vi "Set Event Stop Result_Info.vi"(8 "error in (no error)":errorcluster caption="entrée d'erreur (pas d'erreur)", 10 "Class Popup Result_Info":refnum<user-event>, 11 "Class Popup Result_Info (Virtual) en entrée":refnum<class "Class Popup Result_Info (Virtual).lvclass">) -> (0 "error out":errorcluster caption="sortie d'erreur", 3 "Class Popup Result_Info (Virtual) en sortie":refnum<class "Class Popup Result_Info (Virtual).lvclass">)   [LabVIEW 2020, in "Library Instrument & Equipement.lvlib" / "Library Popup.lvlib" / "Class Popup Result_Info (Virtual).lvclass"]
uses:
  Class Popup Result_Info (Virtual).lvclass
  Class Popup Result_Info (Virtual).lvclass/Class Popup Result_Info (Virtual).ctl
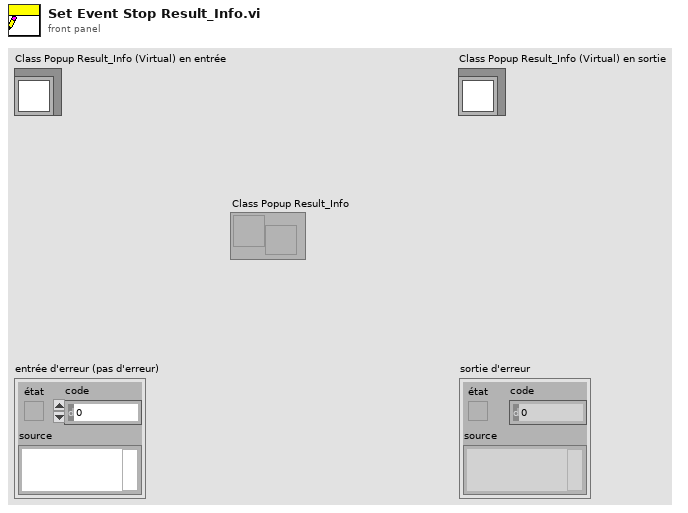
[diagram p1: front panel]
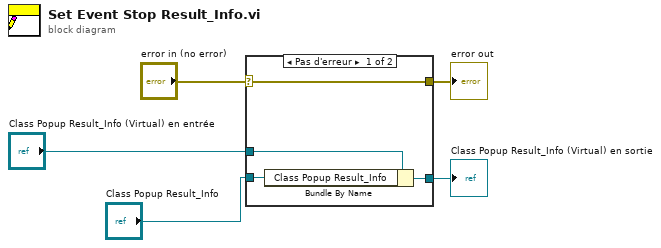
[diagram p0: block diagram]
diagram:
  n1 = case shown="Pas d'erreur" "error in (no error)" {
    selector: "error in (no error)" -> [w9 w10]
    tunnel: [w9 w10] -> w4
    tunnel: [w7 w11] -> w2
    tunnel: "Class Popup Result_Info (Virtual) en entrée" -> [w8 w11]
    tunnel: "Class Popup Result_Info" -> [w6 _]
    frame No Error {
      n2 = Bundle By Name(cluster=w8, "Class Popup Result_Info"=w6) -> (w7:refnum<class "Class Popup Result_Info (Virtual).lvclass">)
    }
    frame Error {
    }
  }
  "error out" <- w4
  "Class Popup Result_Info (Virtual) en sortie" <- w2
